vi "basic case.vi"() -> ()   [LabVIEW 2012]
uses:
  <vilib>/DAQmx/read.llb/DAQmx Read (Analog DBL 1Chan 1Samp).vi
  <vilib>/DAQmx/create/channels.llb/DAQmx Create Channel (AI-Voltage-Basic).vi
panel:
  in  "physical channels":tag
  out "Light Intensity Meter":dbl(knob) scale=0.0..10.0
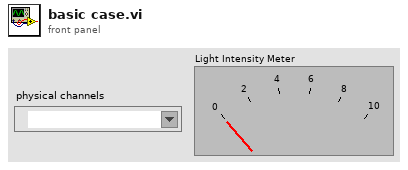
[diagram p1: front panel]
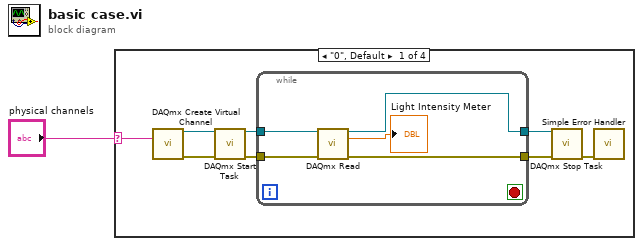
[diagram p0: block diagram]
diagram:
  n1 = case shown="\"0\", Default" "physical channels" {
    selector: "physical channels" -> [w9 _ _ _]
    frame "0", Default {
      n2 = call-poly <vilib>:"DAQmx Create Virtual Channel.vi"("physical channels"=w9) -> ("task out"=w3:refnum<k21>, "error out"=w2:errorcluster)  [unwired: 13 in]
      n3 = call <vilib>:"DAQmx Start Task.vi"("task/channels in"=w3, "error in"=w2) -> ("task out"=w5:refnum<k21>, "error out"=w4:errorcluster)  [unwired: 12 in]
      n4 = while {
        tunnel: w4 -> [w13]
        tunnel: w5 -> [w14]
        tunnel: [w12] -> w6
        tunnel: [w11] -> w8
        stop <- _ stop-if-true
        n5 = call-poly <vilib>:"DAQmx Read.vi"("task/channels in"=w14, "error in"=w13) -> ("task out"=w11:refnum<k21>, "data"=→"Light Intensity Meter":dbl, "error out"=w12:errorcluster)  [unwired: 11 in]
      }
      n6 = call <vilib>:"DAQmx Stop Task.vi"("task/channels in"=w8, "error in"=w6) -> ("error out"=w7:errorcluster)  [unwired: 12 in, 1 out]
      n7 = call <vilib>:"Simple Error Handler.vi"("error in (no error)"=w7) -> ()  [unwired: 4 in, 5 out]
    }
    frame "1".."2" {
    }
    frame "3".."4" {
    }
    frame "5" {
    }
  }
